vi "Replace_Channel_Values.vi"(2 "Channels to replace":string[][](array[string]), 3 "Present Values":string[](array[string]), 4 "Present Channels":string[](array[string])) -> (0 "Merged Row values":string[](array[string]))   [LabVIEW 2010]
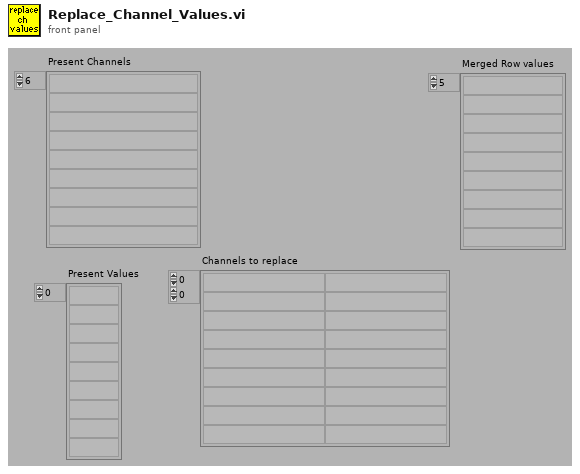
[diagram p1: front panel]
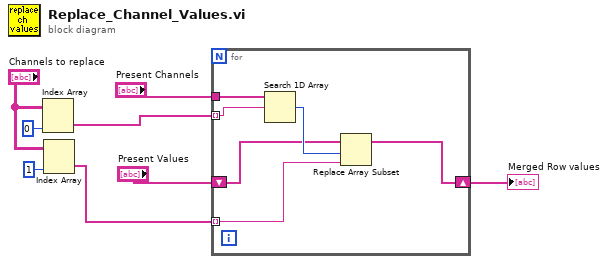
[diagram p0: block diagram]
diagram:
  n1 = Index Array(array="Channels to replace", index (col)=0) -> (element=w1:string[])  [unwired: 1 in]
  n2 = Index Array(array="Channels to replace", index (col)=1) -> (element=w2:string[])  [unwired: 1 in]
  n3 = for {
    tunnel: "Present Channels" -> [w14]
    tunnel: w1 -> [w13] mode=indexing
    shift-right: [w9] -> w6
    shift-left: "Present Values" -> [w11]
    tunnel: w2 -> [w10] mode=indexing
    n4 = Search 1D Array(1D array=w14, element=w13) -> (index of element=w12:i32)  [unwired: 1 out]
    n5 = Replace Array Subset(array=w11, new element=w10, index=w12) -> (w9:string[])
  }
  "Merged Row values" <- w6
